vi "Traffic lights.vi"() -> ()   [LabVIEW 2020]
uses:
  Traffic lights.ctl
panel:
  in  "stop":bool
  out "Green":bool
  out "Yellow":bool
  out "Red":bool
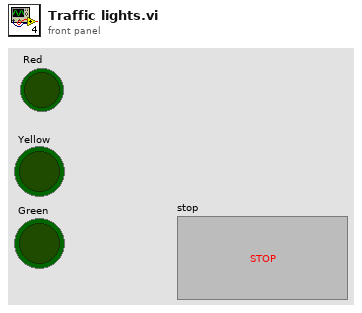
[diagram p1: front panel]
types:
  T1 = typedef "Control 2" = enum16{"Red", "Yellow", "Green"}
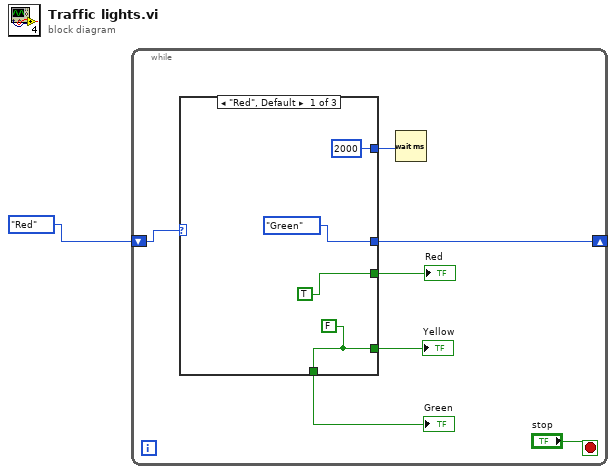
[diagram p0: block diagram]
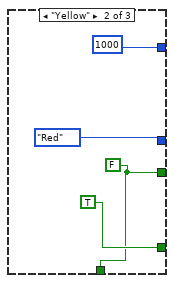
[diagram p2: hidden frame]
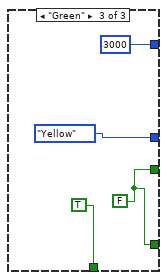
[diagram p3: hidden frame]
diagram:
  n1 = while {
    shift-right: [w7] -> _
    shift-left: Control_2."Red" -> [w8]
    stop <- "stop" stop-if-true
    n2 = case shown="\"Red\", Default" w8 {
      tunnel: [Control_2."Green" Control_2."Red" Control_2."Yellow"] -> w7
      tunnel: [w10 TRUE w18] -> w6
      tunnel: [TRUE w14 w18] -> w5
      tunnel: [w10 w14 TRUE] -> w4
      tunnel: [u32 2000 ("milliseconds to wait") u32 1000 ("milliseconds to wait") u32 3000 ("milliseconds to wait")] -> w3
      frame "Red", Default {
        w10 = FALSE
      }
      frame "Yellow" {
        w14 = FALSE
      }
      frame "Green" {
        w18 = FALSE
      }
    }
    "Red" <- w5
    "Yellow" <- w6
    "Green" <- w4
    n3 = Wait (ms)(milliseconds to wait=w3) -> ()  [unwired: 1 out]
  }
